vi "Discover Plugin Types.vi"(8 "error in (no error)":errorcluster, 11 "CIF_UI in":refnum<class "CIF_UI.lvclass">) -> (0 "error out":errorcluster, 3 "CIF_UI out":refnum<class "CIF_UI.lvclass">)   [LabVIEW 2021, in "CIF_UI.lvclass"]
uses:
  CIF_UI.lvclass
  CIF_UI.lvclass/CIF_UI.ctl
  CIFPluginManager/CIFPluginManager/gRPC/CIF_Manager_Client_Wrapper/CIFManagerClientWrapper.lvlib
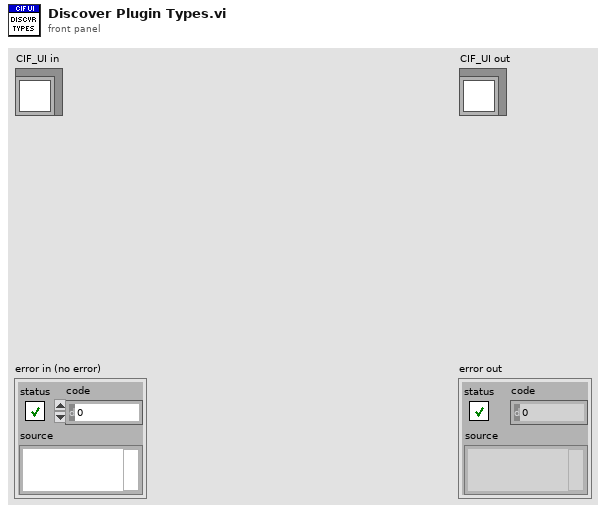
[diagram p1: front panel]
types:
  T1 = typedef "grpc-lvsupport-release.lvlib/grpcId.ctl" = u64
  T2 = typedef "CIF_Manager_client.lvlib/cif_manager_PluginType.ctl" = cluster{"plugin_type":string, "plugin_version":T3}
  T3 = typedef "CIF_Manager_client.lvlib/cif_manager_PluginVersion.ctl" = cluster{"major_version":i32, "minor_version":i32, "fix_version":i32, "build_version":i32}
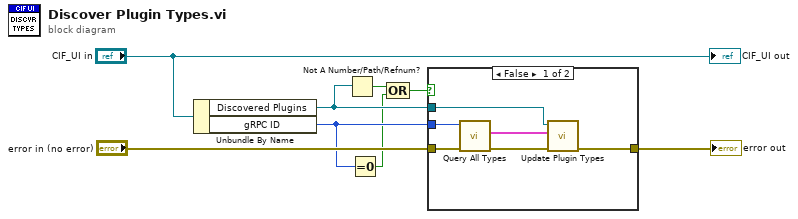
[diagram p0: block diagram]
diagram:
  n1 = Unbundle By Name("CIF_UI in") -> ("Discovered Plugins"=w5:refnum<vi>, "gRPC ID"=w4:T1)
  n2 = Not A Number/Path/Refnum?(number/path/refnum=w5) -> (NaN/Path/Refnum?=w3:bool)
  n3 = Equal To 0?(x=w4) -> (x = 0?=w2:bool)
  n4 = Compound Arithmetic op=OR(w3, w2) -> (w1:bool)
  n5 = case shown="False" w1 {
    tunnel: "error in (no error)" -> [w14 w15]
    tunnel: [w13 w15] -> w7
    tunnel: w4 -> [w10 _]
    tunnel: w5 -> [w9 _]
    frame False {
      n6 = call "Query All Types.vi"("error in"=w14, "gRPC ID in"=w10) -> ("error out"=w12:errorcluster, "plugin_types"=w11:T2[])  [unwired: 7 in, 1 out]
      n7 = call "Update Plugin Types.vi"("error in (no error)"=w12, "plugin_types"=w11, "Plugin Types ref in"=w9) -> ("error out"=w13:errorcluster)  [unwired: 7 in, 1 out]
    }
    frame True {
    }
  }
  "error out" <- w7
  "CIF_UI out" <- "CIF_UI in"
